vi "Character to Code Point.vi"(11 "Character":string) -> (3 "U32 Code Point":u32 format="%.0x", 5 "Byte":u8)   [LabVIEW 2020, in "Stream.lvlib" / "URLPattern.lvclass"]
uses:
  URLPattern.lvclass
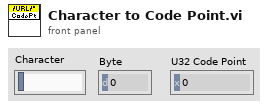
[diagram p1: front panel]
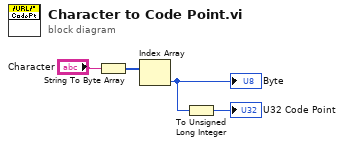
[diagram p0: block diagram]
diagram:
  n1 = String To Byte Array(string="Character") -> (unsigned byte array=w3:u8[])
  n2 = Index Array(array=w3) -> (element=w2:u8)  [unwired: 1 in]
  "Byte" <- w2
  n3 = To Unsigned Long Integer(number=w2) -> (unsigned 32bit integer=→"U32 Code Point":u32)
